vi "Set File Permissions with PDFStamper.vi"(0 "PDFStamper IN":refnum<k24>, 7 "Permissions":T1={"User Password"="", "Owner Password"="", "Printing"=enum."Allow Printing", "Allow Modify Contents"=FALSE, "Allow Copy"=TRUE, "Allow Modify Annotations"=FALSE, "Allow Fill In "=FALSE, "Allow Screen Readers"=TRUE, "Allow Assembly"=FALSE}, 11 "error in (no error)":errorcluster) -> (4 "PDFStamper OUT":refnum<k24>, 15 "error out":errorcluster)   [LabVIEW 2019]
doc: "Version 1.0\nDeveloped by Jean-Marc Simard\nCopyright © 2011, Exaprom Inc.\nAll rights reserved.\nLicense: BSD\n\nWith iTextSharp 4.1.6 (http://itextsharp.sourceforge.net)\nunder Mozilla Public License Version 1.1\n(http://www.mozilla.org/MPL/MPL-1.1.html)"
uses:
  <userlib>/Exaprom PDF/Controls/Initialization Controls/File Permission Parameters.ctl
  C:/Program Files/National Instruments/LabVIEW 2019/user.lib/Exaprom PDF/DLL/itextsharp.dll
  DLL/itextsharp.dll
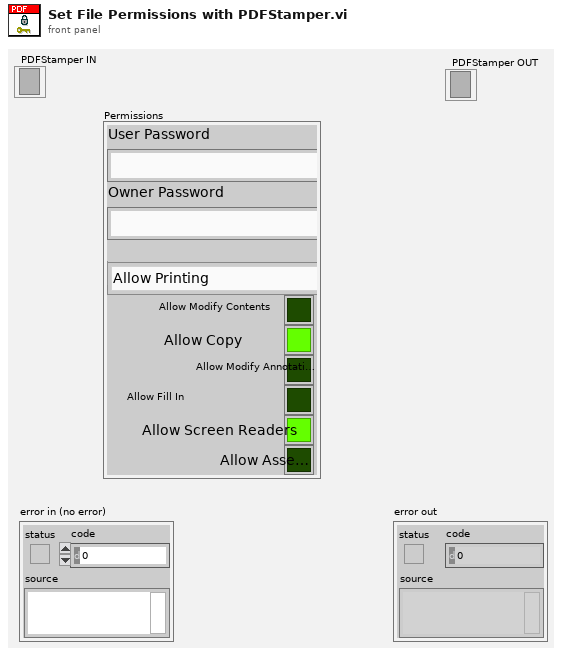
[diagram p1: front panel]
types:
  T1 = typedef "File Permission Parameters.ctl" = cluster{"User Password":string, "Owner Password":string, "Printing":enum16{"Allow Printing", "Allow Degraded Printing", "Don't Allow Printing"}, "Allow Modify Contents":bool, "Allow Copy":bool, "Allow Modify Annotations":bool, "Allow Fill In ":bool, "Allow Screen Readers":bool, "Allow Assembly":bool}
  T2 = cluster{"AllowAssembly":i32, "AllowCopy":i32, "AllowDegradedPrinting":i32, "AllowFillIn":i32, "AllowModifyAnnotations":i32, "AllowModifyContents":i32, "AllowPrinting":i32, "AllowScreenReaders":i32}
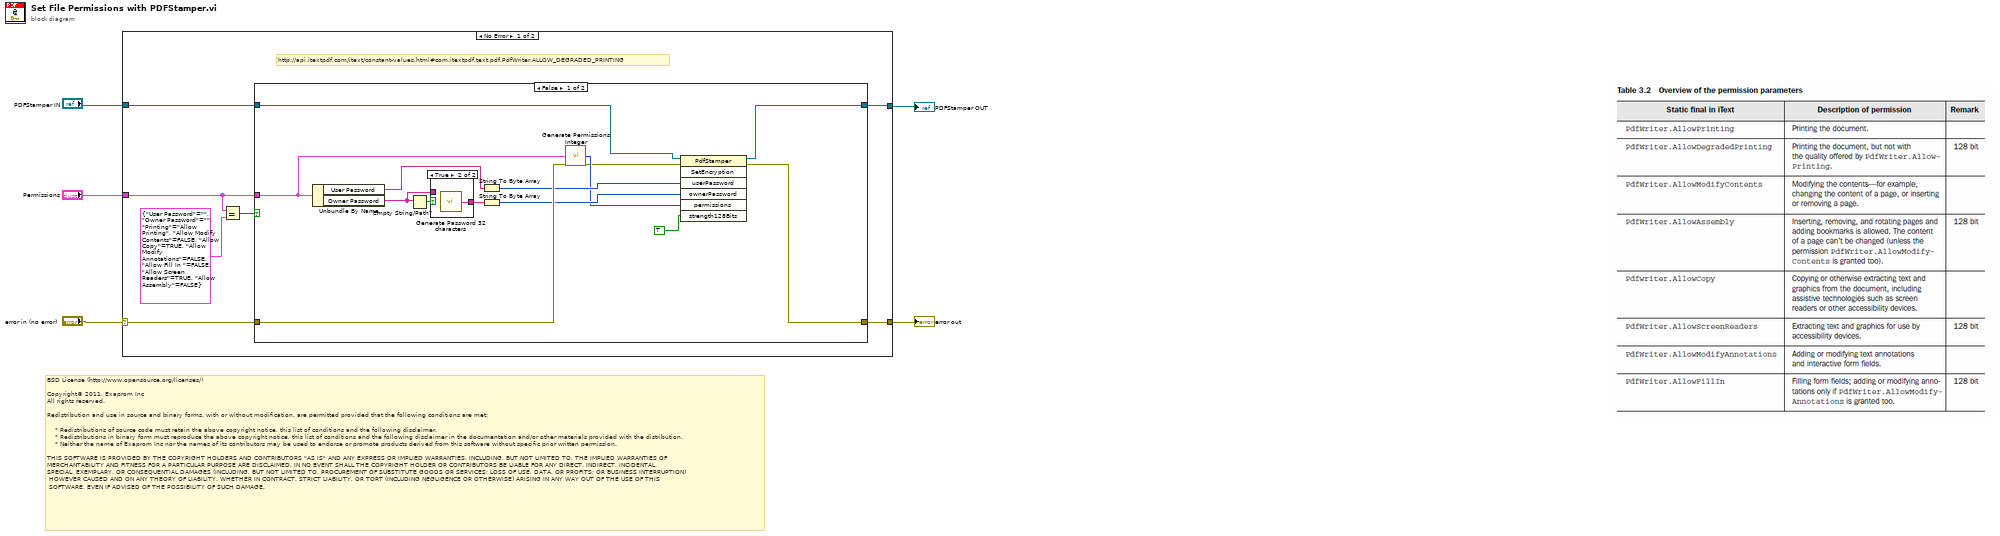
[diagram p0: block diagram]
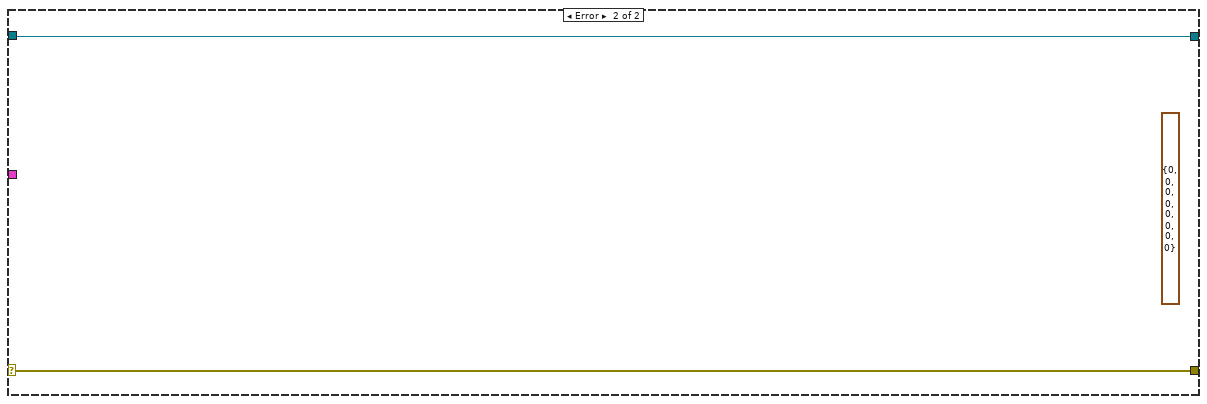
[diagram p4: hidden frame]
diagram:
  # "BSD License (http://www.opensource.org/licenses/)\n\nCopyright© 2011, Exaprom Inc\nAll rights reserved.\n\nRedistribution and use in source and binary forms, with or without modification, are permitted provided that the following conditions are met:\n\n    * Redistributions of source code must retain the above copyright notice, this list of conditions and the following disclaimer.\n    * Redistributions in binary form must reproduce the above copyright notice, this list of conditions and the following disclaimer in the documentation and/or other materials provided with the distribution.\n    * Neither the name of Exaprom Inc nor the names of its contributors may be used to endorse or promote products derived from this software without specific prior written permission.\n\nTHIS SOFTWARE IS PROVIDED BY THE COPYRIGHT HOLDERS AND CONTRIBUTORS \"AS IS\" AND ANY EXPRESS OR IMPLIED WARRANTIES, INCLUDING, BUT NOT LIMITED TO, THE IMPLIED WARRANTIES OF \nMERCHANTABILITY AND FITNESS FOR A PARTICULAR PURPOSE ARE DISCLAIMED. IN NO EVENT SHALL THE COPYRIGHT HOLDER OR CONTRIBUTORS BE LIABLE FOR ANY DIRECT, INDIRECT, INCIDENTAL,\nSPECIAL, EXEMPLARY, OR CONSEQUENTIAL DAMAGES (INCLUDING, BUT NOT LIMITED TO, PROCUREMENT OF SUBSTITUTE GOODS OR SERVICES; LOSS OF USE, DATA, OR PROFITS; OR BUSINESS INTERRUPTION)\n HOWEVER CAUSED AND ON ANY THEORY OF LIABILITY, WHETHER IN CONTRACT, STRICT LIABILITY, OR TORT (INCLUDING NEGLIGENCE OR OTHERWISE) ARISING IN ANY WAY OUT OF THE USE OF THIS\n SOFTWARE, EVEN IF ADVISED OF THE POSSIBILITY OF SUCH DAMAGE."
  n1 = case shown="No Error" "error in (no error)" {
    selector: "error in (no error)" -> [w12 w32]
    tunnel: "PDFStamper IN" -> [w11 w31]
    tunnel: [w6 w31] -> w1
    tunnel: [w10 w32] -> w5
    tunnel: "Permissions" -> [w9 _]
    frame No Error {
      # "http://api.itextpdf.com/itext/constant-values.html#com.itextpdf.text.pdf.PdfWriter.ALLOW_DEGRADED_PRINTING"
      n2 = Equal?(x=w9, y=T1 {"User Password"="", "Owner Password"="", "Printing"=enum."Allow Printing", "Allow Modify Contents"=FALSE, "Allow Copy"=TRUE, "Allow Modify Annotations"=FALSE, "Allow Fill In "=FALSE, "Allow Screen Readers"=TRUE, "Allow Assembly"=FALSE} ("Permissions")) -> (x = y?=w7:bool)
      n3 = case shown="False" w7 {
        tunnel: w12 -> [w26 w30]
        tunnel: w11 -> [w14 w29]
        tunnel: [w18 w30] -> w10
        tunnel: w9 -> [w16 _]
        tunnel: [w13 w29] -> w6
        frame False {
          n4 = Unbundle By Name(w16) -> ("User Password"=w20:string, "Owner Password"=w21:string)
          n5 = Empty String/Path?(string/path=w21) -> (empty?=w23:bool)
          n6 = case shown="True" w23 {
            tunnel: [w27 w28] -> w22
            tunnel: w21 -> [w27 _]
            frame False {
            }
            frame True {
              n7 = call <userlib>:"Generate Password 32 characters.vi"() -> ("Password string"=w28:string)  [unwired: 1 in, 14 out]
            }
          }
          n8 = String To Byte Array(string=w20) -> (unsigned byte array=w24:u8[])
          n9 = String To Byte Array(string=w22) -> (unsigned byte array=w25:u8[])
          n10 = call <userlib>:"Generate Permissions Integer.vi"("Permissions"=w16, "error in (no error)"=w26) -> ("Permissions"=w17:i32, "error out"=w15:errorcluster)  [unwired: 12 out]
          n11 = invoke class="PdfStamper" method="SetEncryption"(reference=w14, error in=w15, "userPassword"=w24, "ownerPassword"=w25, "permissions"=w17, "strength128Bits"=TRUE) -> (reference out=w13:refnum<k24>, error out=w18:errorcluster)  [unwired: 1 in, 5 out]
        }
        frame True {
        }
      }
    }
    frame Error {
      (unwired) T2 {"AllowAssembly"=0, "AllowCopy"=0, "AllowDegradedPrinting"=0, "AllowFillIn"=0, "AllowModifyAnnotations"=0, "AllowModifyContents"=0, "AllowPrinting"=0, "AllowScreenReaders"=0}
    }
  }
  "error out" <- w5
  "PDFStamper OUT" <- w1
